vi "Ventil.vi"() -> ()   [LabVIEW 2011]
panel:
  out "Boolean 3":bool
  out "Boolean 2":bool
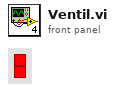
[diagram p1: front panel]
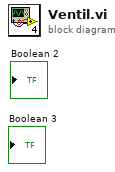
[diagram p0: block diagram]
diagram:
